vi "blue test.vi"   [LabVIEW 2010, in "Bluetooth.lvrbt"]
uses:
  Bluetooth.lvrbt
  <vilib>/NXT/Block Support/NXT_MessageMailbox.ctl
  <vilib>/NXT/Block Support/NXT_InputPort.ctl
  <vilib>/NXT/Dual Mode Library/Sensors/Sonar_cm.vi
  <vilib>/NXT/Dual Mode Library/BT/BlueTooth_Write_Num.vi
  <vilib>/NXT/Dual Mode Library/Sensors/Light_On.vi
types:
  T1 = typedef "NXT_MessageMailbox.ctl" = u8
  T2 = typedef "NXT_InputPort.ctl" = u8
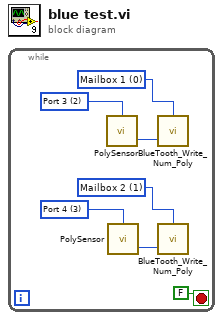
[diagram p0: block diagram]
diagram:
  n1 = while {
    stop <- FALSE stop-if-true
    w2 = T1 1 items=["Mailbox 1", "Mailbox 2", "Mailbox 3", "Mailbox 4", "Mailbox 5", "Mailbox 6", "Mailbox 7", "Mailbox 8", "Mailbox 9", "Mailbox 10"] ("Mailbox")
    w4 = T2 3 items=["Port 1", "Port 2", "Port 3", "Port 4"] ("Port (Port 3)")
    w5 = T1 0 items=["Mailbox 1", "Mailbox 2", "Mailbox 3", "Mailbox 4", "Mailbox 5", "Mailbox 6", "Mailbox 7", "Mailbox 8", "Mailbox 9", "Mailbox 10"] ("Mailbox")
    w7 = T2 2 items=["Port 1", "Port 2", "Port 3", "Port 4"] ("Port (Port 3)")
    n2 = call-poly <vilib>:"PolySensor.vi"("Port (Port 3)"=w7) -> ("Scaled Value"=w6:i16)  [unwired: 2 in, 1 out]
    n3 = call-poly <vilib>:"PolySensor.vi"("Port (Port 4)"=w4) -> ("Distance (cm)"=w3:i16)  [unwired: 2 in, 1 out]
    n4 = call-poly <vilib>:"BlueTooth_Write_Num_Poly.vi"("Message"=w6, "Mailbox"=w5) -> ()  [unwired: 2 in, 1 out]
    n5 = call-poly <vilib>:"BlueTooth_Write_Num_Poly.vi"("Message"=w3, "Mailbox"=w2) -> ()  [unwired: 2 in, 1 out]
  }
